vi "open&auth_ftp.vi"(10 "password":string="5tp010xmd90", 11 "Computer IP":string="localhost") -> (0 "error out":errorcluster, 3 "TCP Network Connection out":T1)   [LabVIEW 2017, in "labview-standard-library.lvlib" / "file-transfer.lvlib"]
uses:
  <vilib>/FTP/ftp0.llb/FTP Session.ctl
  file-transfer.lvlib
  <vilib>/FTP/NI_FTP.lvlib
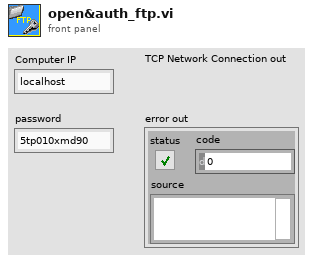
[diagram p1: front panel]
types:
  T1 = typedef "NI_FTP.lvlib/FTP Session.ctl" = refnum<k5>
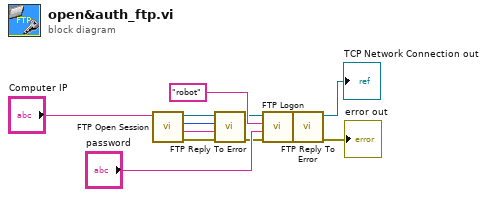
[diagram p0: block diagram]
diagram:
  n1 = call <vilib>:"FTP Open Session.vi"("address"="Computer IP") -> ("error out"=w4:errorcluster, "reply string"=w1:string, "reply code"=w2:i32, "ftp session"=w14:T1)  [unwired: 7 in]
  n2 = call <vilib>:"FTP Reply To Error.vi"("error in (no error)"=w4, "reply string in"=w1, "reply code in"=w2, "ftp session"=w14) -> ("error out"=w3:errorcluster, "ftp session out"=w5:T1)  [unwired: 2 out]
  n3 = call <vilib>:"FTP Logon.vi"("error in (no error)"=w3, "password"="password", "user"="robot", "ftp session"=w5) -> ("error out"=w8:errorcluster, "reply string"=w9:string, "reply code"=w10:i32, "ftp session out"=w11:T1)  [unwired: 4 in]
  n4 = call <vilib>:"FTP Reply To Error.vi"("error in (no error)"=w8, "reply string in"=w9, "reply code in"=w10, "ftp session"=w11) -> ("error out"=→"error out":errorcluster, "ftp session out"=→"TCP Network Connection out":T1)  [unwired: 2 out]
